vi "Configure Math.vi"   [LabVIEW 2013, in "Agilent 90000 Series.lvlib"]
doc: "Configure the math operation."
uses:
  Agilent 90000 Series.lvlib
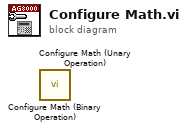
[diagram p0: block diagram]
diagram:
  n1 = call "Configure Math (Binary Operation).vi"() -> ()  [unwired: 14 in, 2 out]
  n2 = call "Configure Math (Unary Operation).vi"() -> ()  [unwired: 14 in, 2 out]
